vi "MainProgram.vi"() -> ()   [LabVIEW 2018]
uses:
  <vilib>/userdefined/High Color/IMAQdx.ctl
  <vilib>/robotics/Navigation/shared/MapNode/OccupancyGridNode/NI_Robotics_OccupancyGridMapNode.lvclass
  C:/Program Files (x86)/National Instruments/LabVIEW 2018/vi.lib/robotics/Navigation/shared/MapNode/AbstractAstarNode/NI_Robotics_AbstractAstarNode.lvclass
  <vilib>/robotics/Navigation/shared/WorldMap/OccupancyGridWorldMap/NI_Robotics_OccupancyGridWorldMap.lvclass
  C:/Program Files (x86)/National Instruments/LabVIEW 2018/vi.lib/robotics/Navigation/shared/WorldMap/AbstractWorldMap/NI_Robotics_AbstractWorldMap.lvclass
  <vilib>/robotics/Navigation/NI_Robotics_Navigation .lvlib
panel:
  out "Position (mm)":cluster{"X":dbl, "Y":dbl, "Theta":dbl}
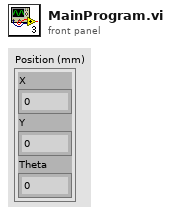
[diagram p1: front panel]
types:
  T1 = typedef "IMAQdx.ctl" = refnum<k21>
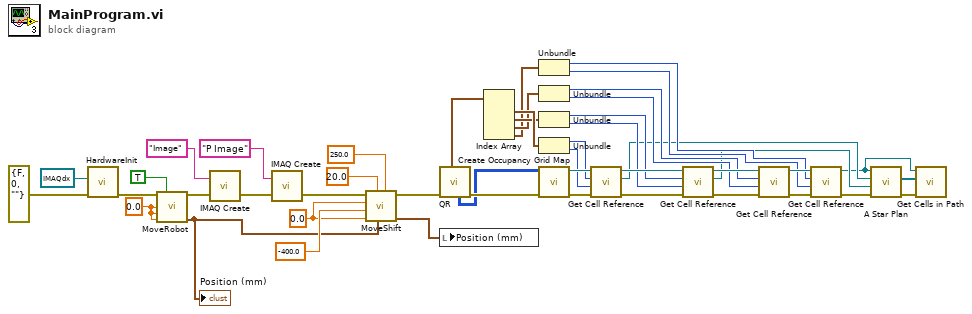
[diagram p0: block diagram]
diagram:
  w34 = 0.0 ("theta")
  w43 = 0.0 ("x (mm/s)")
  n1 = call "HardwareInit.vi"("Error/Flow In"=errorcluster {"status"=FALSE, "code"=0, "source"=""}, "Session In"=T1 refnum) -> ("error out"=w44:errorcluster)  [unwired: 8 in, 1 out]
  n2 = call "MoveRobot.vi"("Error/Flow In"=w44, "Reset"=TRUE, "x (mm/s)"=w43, "y (mm/s)"=w43, "theta (rad/s)"=w43) -> ("Error/Flow Out"=w41:errorcluster, "Position"=w1:cluster{"X":dbl, "Y":dbl, "Theta":dbl})  [unwired: 9 in]
  "Position (mm)" <- w1
  n3 = call "IMAQ Create"("Image Name"="Image", "error in (no error)"=w41) -> ("error out"=w39:errorcluster)  [unwired: 3 in, 1 out]
  n4 = call "IMAQ Create"("Image Name"="P Image", "error in (no error)"=w39) -> ("error out"=w37:errorcluster)  [unwired: 3 in, 1 out]
  n5 = call "MoveShift.vi"("max speed"=250.0, "Position"=w1, "Precision"=20.0, "theta"=w34, "y shift"=-400.0, "x shift"=w34, "Error/Flow In"=w37) -> ("Position Out"=w35:cluster{"X":dbl, "Y":dbl, "Theta":dbl}, "Error/Flow Out"=w31:errorcluster)  [unwired: 3 in]
  n6 = call "QR.vi"("error in"=w31) -> ("error out"=w30:errorcluster, "G"=w29:i32[][], "Control Points"=w28:cluster{"third_x":i32, "third_y":i32}[])  [unwired: 3 in, 5 out]
  n7 = local write "Position (mm)"(w35) -> ()
  n8 = Index Array(array=w28) -> (element #1=w27:cluster{"third_x":i32, "third_y":i32}, element #2=w16:cluster{"third_x":i32, "third_y":i32}, element #3=w11:cluster{"third_x":i32, "third_y":i32}, element #4=w10:cluster{"third_x":i32, "third_y":i32})  [unwired: 4 in]
  n9 = Unbundle(w10) -> ("third_x"=w9:i32, "third_y"=w8:i32)
  n10 = Unbundle(w11) -> ("third_x"=w13:i32, "third_y"=w12:i32)
  n11 = Unbundle(w16) -> ("third_x"=w15:i32, "third_y"=w14:i32)
  n12 = Unbundle(w27) -> ("third_x"=w18:i32, "third_y"=w17:i32)
  n13 = call <vilib>:"Create Occupancy Grid Map.vi"("error in (no error)"=w30, "occupancy grid"=w29) -> ("error out"=w26:errorcluster, "map reference out"=w25:refnum<data-value>)  [unwired: 8 in]
  n14 = call <vilib>:"Get Cell Reference.vi"("error in (no error)"=w26, "y"=w17, "x"=w18, "map reference in"=w25) -> ("error out"=w24:errorcluster, "cell reference"=w7:refnum<data-value>, "map reference out"=w23:refnum<data-value>)  [unwired: 4 in, 1 out]
  n15 = call <vilib>:"Get Cell Reference.vi"("error in (no error)"=w24, "y"=w14, "x"=w15, "map reference in"=w23) -> ("error out"=w22:errorcluster, "cell reference"=w6:refnum<data-value>, "map reference out"=w21:refnum<data-value>)  [unwired: 4 in, 1 out]
  n16 = call <vilib>:"Get Cell Reference.vi"("error in (no error)"=w22, "y"=w12, "x"=w13, "map reference in"=w21) -> ("error out"=w19:errorcluster, "map reference out"=w20:refnum<data-value>)  [unwired: 4 in, 2 out]
  n17 = call <vilib>:"Get Cell Reference.vi"("error in (no error)"=w19, "y"=w8, "x"=w9, "map reference in"=w20) -> ("error out"=w5:errorcluster, "map reference out"=w2:refnum<data-value>)  [unwired: 4 in, 2 out]
  n18 = call <vilib>:"A Star Plan.vi"("error in (no error)"=w5, "goal reference"=w6, "start reference"=w7, "map reference in"=w2) -> ("error out"=w4:errorcluster, "path references"=w3:refnum<data-value>[])  [unwired: 4 in, 2 out]
  n19 = call <vilib>:"Get Cells in Path.vi"("error in (no error)"=w4, "path references"=w3, "map reference in"=w2) -> ()  [unwired: 5 in, 4 out]
